vi "Get 负载电压.vi"(11 "EPEVER-MPPT in":refnum<class "EPEVER-MPPT.lvclass">) -> (2 "负载电压":refnum<vi>, 3 "EPEVER-MPPT out":refnum<class "EPEVER-MPPT.lvclass">)   [LabVIEW 2016, in "EPEVER-MPPT.lvlib" / "EPEVER-MPPT.lvclass"]
uses:
  EPEVER-MPPT.lvclass
  EPEVER-MPPT.lvclass/EPEVER-MPPT.ctl
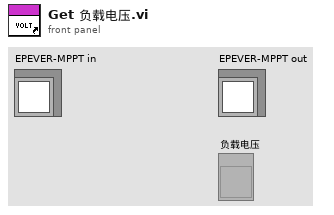
[diagram p1: front panel]
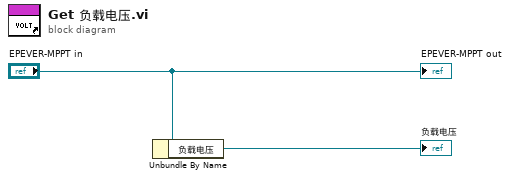
[diagram p0: block diagram]
diagram:
  n1 = Unbundle By Name("EPEVER-MPPT in") -> ("负载电压"=→"负载电压":refnum<vi>)
  "EPEVER-MPPT out" <- "EPEVER-MPPT in"
